vi "PH_BlackBox.PC Calc Position.vi"(0 "i ref in":refnum<vi>, 5 "error in (no error)":errorcluster) -> (14 "i ref out":refnum<vi>, 19 "error out":errorcluster)   [LabVIEW 2014, in "PH_BlackBox.lvlib"]
doc: "Within this VI the current position is calculated and - if it has changed - written to own attributes and published as DIM service."
uses:
  PH_BlackBox.lvlib
  PH_Basics/PH_StatusHandler/PH_StatusHandler.Status.ctl
  PH_Basics/PH_StatusHandler/PH_StatusHandler.lvlib
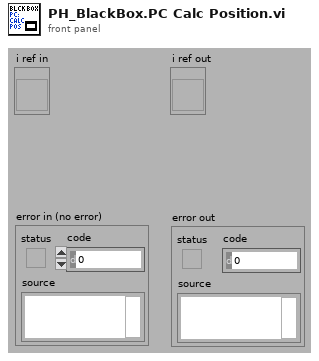
[diagram p1: front panel]
types:
  T1 = enum8{"Enabled", "Disabled", "Disabled and Grayed Out"}
  T2 = typedef "PH_StatusHandler.lvlib/PH_StatusHandler.Status.ctl" = i16
  T3 = typedef "PH_BlackBox.lvlib/PH_BlackBox.i attribute.ctl" = cluster{"BB Remote Controlled?":bool, "GUI Refs":T4, "Position IN":T2, "Position OUT":T2, "BB Remote Controlled by other Instance?":bool, "Recipient":string, "Number":i32, "Caption Move":string, "Caption Out":string, "Caption In":string}
  T4 = typedef "PH_BlackBox.lvlib/PH_BlackBox.GUI Refs.ctl" = cluster{"MOVE IN":refnum<vi>, "MOVE":refnum<vi>, "IN":refnum<vi>, "OUT":refnum<vi>, "REMOTE":refnum<vi>, "GUI-Knob Move":refnum<vi>, "GUI-Knob Move in":refnum<vi>, "POWER ON":refnum<vi>, "Delete":refnum<vi>, "Function Textfield":refnum<vi>}
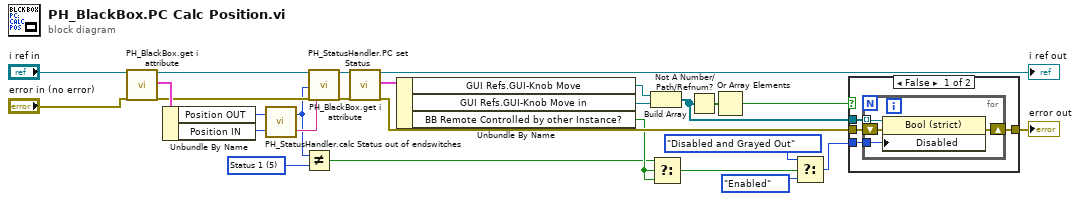
[diagram p0: block diagram]
diagram:
  w10 = T2 5 items=["no info", "off/false/out", "on/true/in", "Failure", "Alarm", "Status 1", "Status 2", "Status 3"] ("y")
  n1 = call "PH_BlackBox.get i attribute.vi"("i ref in"="i ref in", "error in (no error)"="error in (no error)") -> ("i ref out"=w25:refnum<vi>, "i attribute"=w27:T3, "error out"=w26:errorcluster)  [unwired: 15 in]
  n2 = Unbundle By Name(w27) -> ("Position OUT"=w8:T2, "Position IN"=w7:T2)
  n3 = call "PH_StatusHandler.calc Status out of endswitches.vi"("Status Input 2: \"True\""=w7, "Status Input 1: \"False\""=w8) -> ("Further Information"=w6:string, "Status Output"=w5:T2)
  n4 = Not Equal?(x=w5, y=w10) -> (x != y?=w9:bool)
  n5 = call "PH_StatusHandler.PC set Status.vi"("i ref in"=w25, "Status"=w5, "error in (no error)"=w26, "Tip Strip"=w6) -> ("i ref out"=w4:refnum<vi>, "error out"=w3:errorcluster)  [unwired: 14 in]
  n6 = call "PH_BlackBox.get i attribute.vi"("i ref in"=w4, "error in (no error)"=w3) -> ("i ref out"=→"i ref out":refnum<vi>, "i attribute"=w16:T3, "error out"=w15:errorcluster)  [unwired: 15 in]
  n7 = Unbundle By Name(w16) -> ("GUI Refs.GUI-Knob Move"=w22:refnum<vi>, "GUI Refs.GUI-Knob Move in"=w13:refnum<vi>, "BB Remote Controlled by other Instance?"=w11:bool)
  n8 = Build Array(w22, w13) -> (w19:refnum<vi>[])
  n9 = Select(t=w9, s=w11, f=w11) -> (s? t:f=w12:bool)
  n10 = Not A Number/Path/Refnum?(number/path/refnum=w19) -> (NaN/Path/Refnum?=w21:bool[])
  n11 = Or Array Elements(Boolean array=w21) -> (logical OR=w20:bool)
  n12 = Select(t=T1."Disabled and Grayed Out" ("Disabled"), s=w12, f=T1."Enabled" ("Disabled")) -> (s? t:f=w18:T1)
  n13 = case shown="False" w20 {
    tunnel: w19 -> [w31 _]
    tunnel: w18 -> [w30 _]
    tunnel: w15 -> [w29 w36]
    tunnel: [w28 w36] -> w14
    frame False {
      n14 = for {
        shift-right: [w34] -> w28
        shift-left: w29 -> [w35]
        tunnel: w31 -> [w33] mode=indexing
        tunnel: w30 -> [w32]
        n15 = property class="Bool (strict)"(reference=w33, error in=w35, "Disabled"=w32) -> (error out=w34:errorcluster)  [unwired: 1 out]
      }
    }
    frame True {
    }
  }
  "error out" <- w14
